vi "FPGA Read - Boolean.vi"(8 "error in (no error)":errorcluster, 10 "Indicator":T1, 11 "FPGA Session In":refnum<class "Firmware Independent PID Interface.lvclass">) -> (0 "error out":errorcluster, 2 "Value":bool, 3 "FPGA Session Out":refnum<class "Firmware Independent PID Interface.lvclass">)   [LabVIEW 2010, in "Firmware Independent PID Interface.lvclass"]
doc: "Reads a boolean value from a given indicator or control."
uses:
  Firmware Independent PID Interface.lvclass
  TypeDefs/IndicatorBool.ctl
  <vilib>/rvi/DataTransferAndStorage/Container/Common/niFpgaDataTypeControl.ctl
  <userlib>/_FPGA Interface Advanced Tools/FPGA Interface Base/FPGA Interface Base.lvclass/FPGA Interface Base.ctl
  <vilib>/Utility/error.llb/Error Cluster From Error Code.vi
  <userlib>/_FPGA Interface Advanced Tools/FPGA Interface Base/Accessors/FPGA Read Session.vi
  <userlib>/_FPGA Interface Advanced Tools/FPGA Interface Wrapper/FPGA Interface Wrapper.lvlib
  <userlib>/_FPGA Interface Advanced Tools/FPGA Interface Base/FPGA Interface Base.lvclass
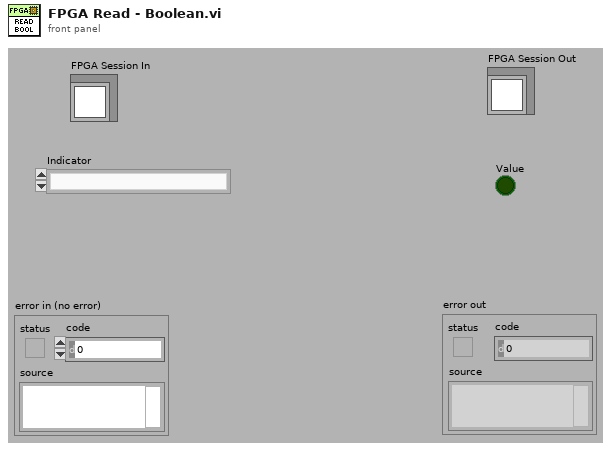
[diagram p1: front panel]
types:
  T1 = typedef "Firmware Independent PID Interface.lvclass/IndicatorBool.ctl" = enum16{""}
  T2 = typedef "niFpgaDataTypeControl.ctl" = enum32{"Boolean", "I8", "I16", "I32", "I64", "U8", "U16", "U32", "U64", "FXP", "CustomControl"}
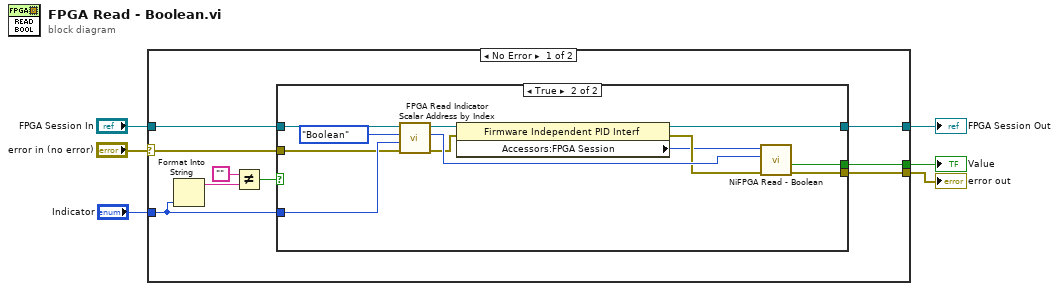
[diagram p0: block diagram]
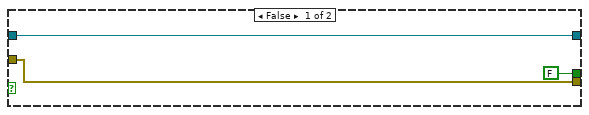
[diagram p2: hidden frame]
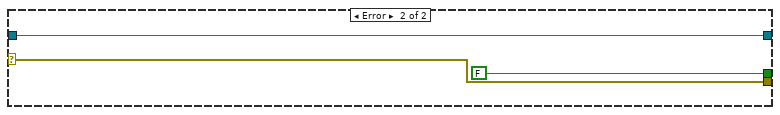
[diagram p3: hidden frame]
diagram:
  n1 = case shown="No Error" "error in (no error)" {
    selector: "error in (no error)" -> [w7 w33]
    tunnel: [w10 w33] -> w5
    tunnel: [w8 w31] -> w2
    tunnel: [w9 FALSE] -> w4
    tunnel: "FPGA Session In" -> [w13 w31]
    tunnel: "Indicator" -> [w11 _]
    frame No Error {
      n2 = Format Into String(w11) -> (resulting string=w15:string)  [unwired: 3 in, 1 out]
      n3 = Not Equal?(x="", y=w15) -> (x != y?=w12:bool)
      n4 = case shown="True" w12 {
        tunnel: [w16 w21] -> w10
        tunnel: [w17 w22] -> w8
        tunnel: [FALSE w30] -> w9
        tunnel: w13 -> [w17 w23]
        tunnel: w11 -> [_ w20]
        tunnel: w7 -> [w16 w19]
        frame False {
        }
        frame True {
          n5 = call <userlib>:"FPGA Read Indicator Scalar Address by Index.vi"("error in (no error)"=w19, "index"=w20, "Data Type"=niFpgaDataTypeControl."Boolean", "FPGA Interface Base in"=w23) -> ("error out"=w27:errorcluster, "Address"=w28:u32, "FPGA Interface Base out"=w26:refnum<class "Firmware Independent PID Interface.lvclass">)  [unwired: 4 in, 1 out]
          n6 = property class="Firmware Independent PID Interf"(reference=w26, error in=w27) -> (reference out=w22:refnum<class "Firmware Independent PID Interface.lvclass">, error out=w25:errorcluster, "Accessors:FPGA Session"=w24:u32)
          n7 = call <userlib>:"NiFPGA Read - Boolean.vi"("error in (no error)"=w25, "Indicator"=w28, "Session"=w24) -> ("error out"=w21:errorcluster, "Boolean"=w30:bool)  [unwired: 6 in, 1 out]
        }
      }
    }
    frame Error {
    }
  }
  "error out" <- w5
  "Value" <- w4
  "FPGA Session Out" <- w2
